vi "V-Meter Configure (2182A).vi"(8 "error in (no error)":errorcluster, 11 "VISA resource name in":refnum<visa-resource-name>) -> (0 "error out":errorcluster, 3 "VISA resource name out":refnum<visa-resource-name>)   [LabVIEW 2016, in "Hall Effect Library.lvlib"]
uses:
  Hall Effect Library.lvlib
  Global Variables/Test Settings.vi
  <instrlib>/Keithley 2182A/Public/Configure/Configure DC Volts.vi
  <instrlib>/Keithley 2182A/Keithley 2182A.lvlib
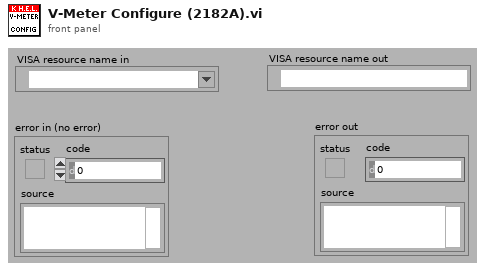
[diagram p1: front panel]
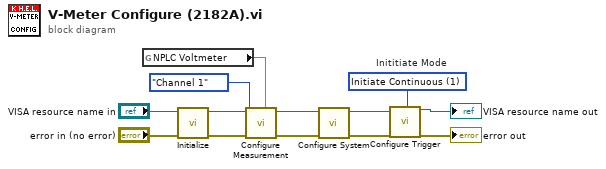
[diagram p0: block diagram]
diagram:
  w7 = i16 1 items=["Don't Initiate"=-1, "Initiate Single"=0, "Initiate Continuous"=1]  # Inititiate Mode
  n1 = global read "Test Settings.vi" "NPLC Voltmeter"() -> (w5:dbl)
  n2 = call <instrlib>:"Initialize.vi"("error in (no error)"="error in (no error)", "VISA resource name"="VISA resource name in") -> ("error out"=w12:errorcluster, "VISA resource name out"=w13:refnum<visa-resource-name>)  [unwired: 3 in, 5 out]
  n3 = call-poly <instrlib>:"Configure Measurement.vi"("NPLC (1)"=w5, "error in"=w12, "Channel (Channel 1)"=enum16{"Channel 1", "Channel 2"}."Channel 1", "VISA resource name"=w13) -> ("error out"=w3:errorcluster, "VISA resource name out"=w4:refnum<visa-resource-name>)  [unwired: 2 in, 4 out]
  n4 = call <instrlib>:"Configure System.vi"("error in"=w3, "VISA resource name"=w4) -> ("error out"=w2:errorcluster, "VISA resource name out"=w1:refnum<visa-resource-name>)  [unwired: 2 in, 6 out]
  n5 = call <instrlib>:"Configure Trigger.vi"("VISA resource name"=w1, "error in"=w2, "Inititiate Mode (Init Continuous)"=w7) -> ("VISA resource name out"=→"VISA resource name out":refnum<visa-resource-name>, "error out"=→"error out":errorcluster)  [unwired: 6 in, 9 out]
